vi "ADC_modify_Ch_and_spans.vi"(0 "Ch & spans":T1[](array[typedef])=[{"high limit (10V)"=10.0, "low limit (-10V)"=-10.0, "Ch No"=0, "Var name"="", "Use Latest Calib"=FALSE}] {"low limit (-10V)" format="%.3f"; "high limit (10V)" format="%.3f"}) -> (1 "group channel settings":T2(array[cluster]) {"scale offset" format="%.2f"; "scale multiplier" format="%.2f"; "gain" format="%.2f"; "range" format="%.2f"; "lower input limits" format="%.2f"; "upper input limits" format="%.2f"}, 2 "Modified Ch & spans":T1[](array[typedef]) {"low limit (-10V)" format="%.3f"; "high limit (10V)" format="%.3f"})   [LabVIEW 2010]
uses:
  Controls/Ch_and_Spans.ctl
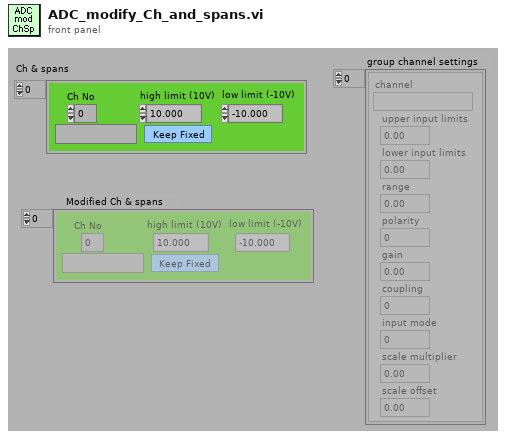
[diagram p1: front panel]
types:
  T1 = typedef "Ch_and_Spans.ctl" = cluster{"high limit (10V)":sgl, "low limit (-10V)":sgl, "Ch No":i16, "Var name":string, "Use Latest Calib":bool}
  T2 = cluster{"channel":string, "upper input limits":sgl, "lower input limits":sgl, "range":sgl, "polarity":u16, "gain":sgl, "coupling":u16, "input mode":u16, "scale multiplier":dbl, "scale offset":dbl}[]
  T3 = cluster{"channel":string, "upper input limits":sgl, "lower input limits":sgl, "range":sgl, "polarity":u16, "gain":sgl, "coupling":u16, "input mode":u16, "scale multiplier":dbl, "scale offset":dbl}
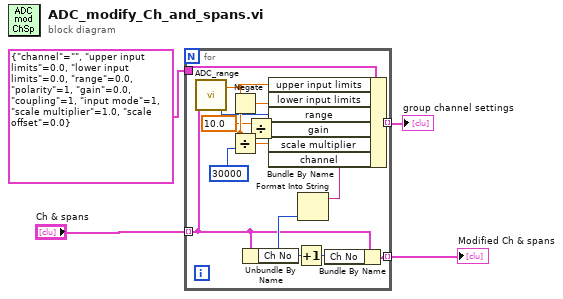
[diagram p0: block diagram]
diagram:
  n1 = for {
    tunnel: "Ch & spans" -> [w13] mode=indexing
    tunnel: [w16] -> w2 mode=indexing
    tunnel: [w15] -> w3 mode=indexing
    tunnel: T3 {"channel"="", "upper input limits"=0.0, "lower input limits"=0.0, "range"=0.0, "polarity"=1, "gain"=0.0, "coupling"=1, "input mode"=1, "scale multiplier"=1.0, "scale offset"=0.0} -> [w14]
    n2 = call "ADC_range.vi"("Channels & Spans"=w13) -> ("Range Code"=w5:i32, "MaxABS( Voltage)"=w7:dbl)  [unwired: 3 out]
    n3 = Negate(x=w7) -> (-x=w12:dbl)
    n4 = Divide(x=w7, y=i16 30000 ("full scale bits")) -> (x/y=w10:dbl)
    n5 = Unbundle By Name(w13) -> ("Ch No"=w18:i16)
    n6 = Divide(x=sgl 10.0, y=w7) -> (x/y=w8:dbl)
    n7 = Increment(x=w18) -> (x+1=w17:i16)
    n8 = Format Into String(w18) -> (resulting string=w11:string)  [unwired: 3 in, 1 out]
    n9 = Bundle By Name(cluster=w14, "upper input limits"=w7, "lower input limits"=w12, "range"=w5, "gain"=w8, "scale multiplier"=w10, "channel"=w11) -> (w15:T3)
    n10 = Bundle By Name(cluster=w13, "Ch No"=w17) -> (w16:T1)
  }
  "group channel settings" <- w3
  "Modified Ch & spans" <- w2
